vi "Dynamixel XL320 Read All Data From Motor(s).vi"(8 "Error in":errorcluster, 9 "Motor ID List":u8[](array[numeric]), 10 "Force Baud Rate (True)":bool=TRUE, 11 "VISA resource name":refnum<visa-resource-name>) -> (0 "error out":errorcluster, 2 "Motor Properties":string[][](table))   [LabVIEW 2015]
doc: "This example shows how to collect all of the available data from a Dynamixel motor."
uses:
  <instrlib>/Dynamixel XL320/Public/Motor Operation/Low Level/XL320_Baud Setting.ctl
  <instrlib>/Dynamixel XL320/Dynamixel XL320.lvlib
panel:
  in  "Baud rate (57600 bps)":T1=34 items=["1,000,000 bps"=1, "500,000 bps"=3, "400,000 bps"=4, "250,000 bps"=7, "200,000 bps"=9, "115200 bps"=16, "57600 bps"=34, "19200 bps"=103, "9600 bps"=207]
  in  "Timeout (30 msec)":u32=30
  # "(c) 2011-2012  National Instruments.  ALL RIGHTS RESERVED."
  # "Input the motor IDs of all of the motors connected in the chain that you want to query.  Then run the VI."
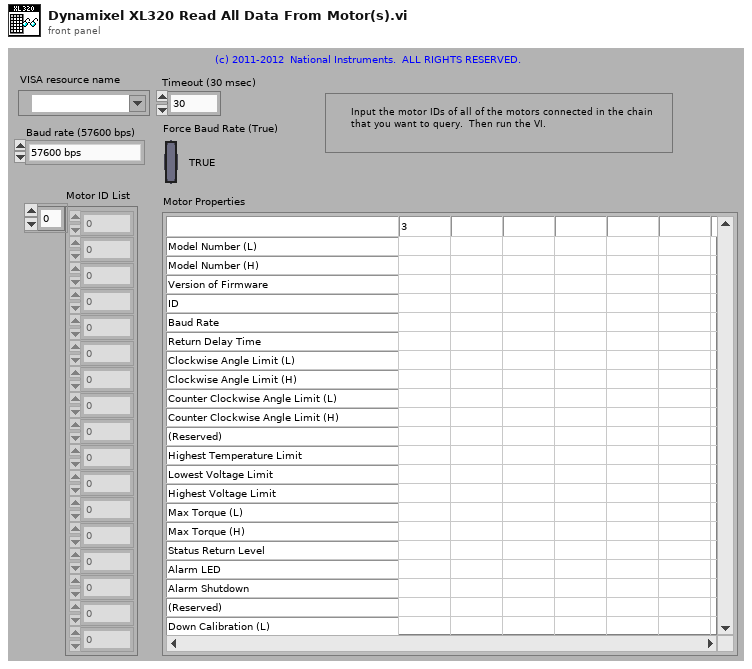
[diagram p1: front panel]
types:
  T1 = typedef "Dynamixel XL320.lvlib/XL320_Baud Setting.ctl" = u8
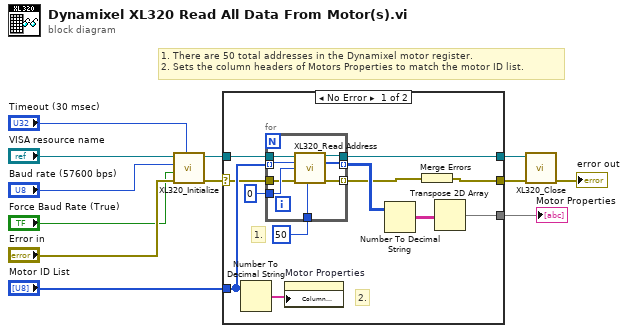
[diagram p0: block diagram]
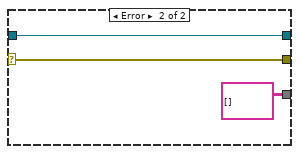
[diagram p2: hidden frame]
diagram:
  # "1. There are 50 total addresses in the Dynamixel motor register.\n2. Sets the column headers of Motors Properties to match the motor ID list."
  n1 = call <instrlib>:"XL320_Initialize.vi"("Timeout (30 msec)"="Timeout (30 msec)", "error in (no error)"="Error in", "Force Baud Rate (True)"="Force Baud Rate (True)", "Baud rate (57600 bps)"="Baud rate (57600 bps)", "VISA resource name"="VISA resource name") -> ("error out"=w4:errorcluster, "VISA resource name out"=w5:refnum<visa-resource-name>)  [unwired: 5 in]
  n2 = case shown="No Error" w4 {
    selector: w4 -> [w14 w35]
    tunnel: [w16 w35] -> w2
    tunnel: [w23 w34] -> w3
    tunnel: w5 -> [w24 w34]
    tunnel: "Motor ID List" -> [w21 _]
    tunnel: [w18 string[][] []] -> w12
    frame No Error {
      # "2."
      # "1."
      n3 = Number To Decimal String(number=w21) -> (decimal integer string=w22:string[])  [unwired: 1 in]
      n4 = for {
        tunnel: w24 -> [w29]
        tunnel: [w32] -> w23
        tunnel: w21 -> [w28] mode=indexing
        tunnel: [w30] -> w17 mode=indexing
        tunnel: [w31] -> w20 mode=indexing
        tunnel: u8 0 ("Address number (dec)") -> [w27]
        tunnel: w14 -> [w25]
        tunnel: u8 50 ("Number of Addresses to read (1)") -> [w26]
        n5 = call <instrlib>:"XL320_Read Address.vi"("VISA resource name"=w29, "Motor ID (0)"=w28, "Address number (0)"=w27, "Number of Addresses to read (1)"=w26, "Error in (no error)"=w25) -> ("VISA resource name Out"=w32:refnum<visa-resource-name>, "Data Read"=w31:u8[], "error out"=w30:errorcluster)  [unwired: 7 in, 1 out]
      }
      n6 = property on="Motor Properties" class="Tbl (strict)"("Column Headers[]"=w22) -> ()  [unwired: 2 in, 2 out]
      n7 = Number To Decimal String(number=w20) -> (decimal integer string=w19:string[][])  [unwired: 1 in]
      n8 = Merge Errors(w17) -> (w16:errorcluster)
      n9 = Transpose 2D Array(2D array=w19) -> (transposed array=w18:string[][])
    }
    frame Error {
    }
  }
  "Motor Properties" <- w12
  n10 = call <instrlib>:"XL320_Close.vi"("error in (no error)"=w2, "VISA resource name"=w3) -> ("error out"=→"error out":errorcluster)  [unwired: 9 in]
